vi "Post action control.vi"(1 "Action":u16(ring)=4 items=["Clear DAQ Tasks", "Check Temperature", "Check Field Value", "Wait", "Do Nothing"], 2 "Scan Parameters":T1={"DAQ Channel"=1, "Label"="\nappliedVsg=", "Scaled low"=-0.1, "Scaled high"=0.1, "Start"=-0.32, "End"=0.42, "Step"=0.002, "Scale?"=FALSE} {"Step" format="%#_6p"; "End" format="%#_6p"; "Start" format="%#_6p"; "Scaled high" format="%#_6p"; "Scaled low" format="%#_6p"}, 3 "Index":dbl=370.0) -> (0 "Out":u16(ring)=4 items=["Clear DAQ Tasks", "Check Temperature", "Check Field Value", "Do Nothing"])   [LabVIEW 2013]
uses:
  <userlib>/LevyLab/PPMS_VIs/Lockin-4461_MultiChannel - IV 3.0 globals.vi
panel:
  in  "target temperature":dbl=0.07
  in  "milliseconds to wait":u32=5000
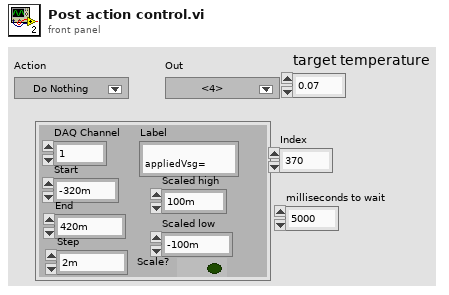
[diagram p1: front panel]
types:
  T1 = cluster{"DAQ Channel":i32, "Label":string, "Scaled low":dbl, "Scaled high":dbl, "Start":dbl, "End":dbl, "Step":dbl, "Scale?":bool}
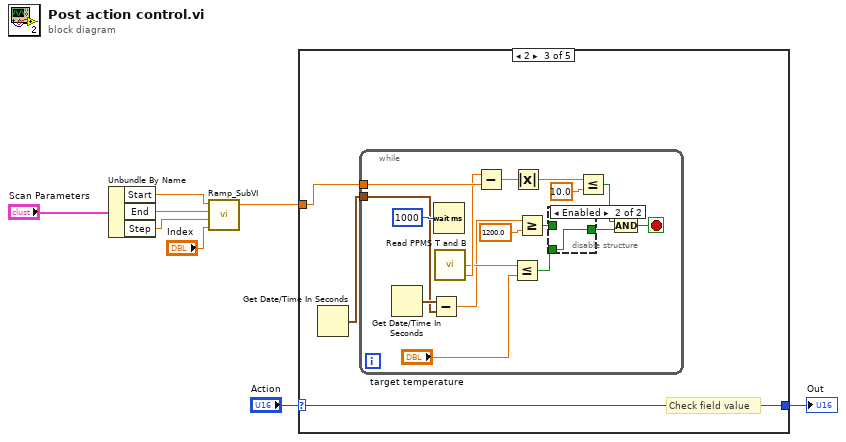
[diagram p0: block diagram]
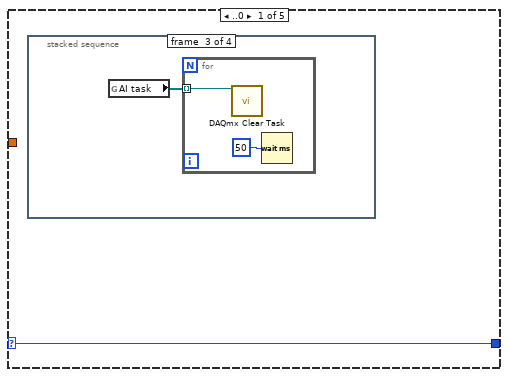
[diagram p2: hidden frame]
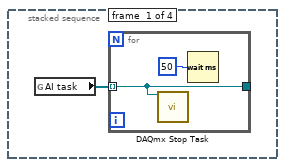
[diagram p3: hidden frame]
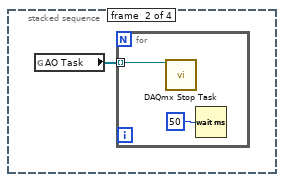
[diagram p4: hidden frame]
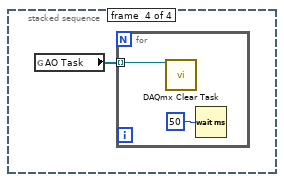
[diagram p5: hidden frame]
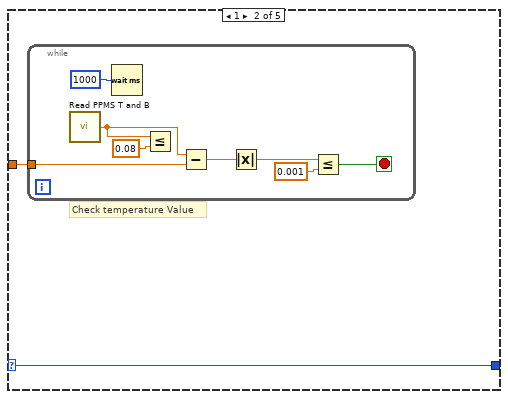
[diagram p6: hidden frame]
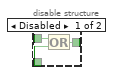
[diagram p7: hidden frame]
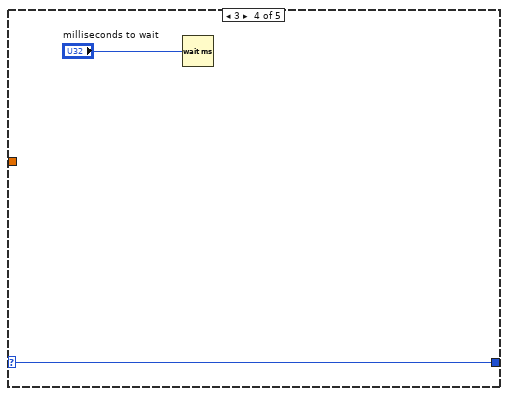
[diagram p8: hidden frame]
diagram:
  n1 = Unbundle By Name("Scan Parameters") -> ("Start"=w5:dbl, "End"=w4:dbl, "Step"=w3:dbl)
  n2 = call <userlib>:"Ramp_SubVI.vi"("index"="Index", "step"=w3, "end"=w4, "start"=w5) -> ("Numeric"=w7:dbl)  [unwired: 1 in, 1 out]
  n3 = case shown="2" "Action" {
    tunnel: w7 -> [_ w23 w34 _ _]
    selector: "Action" -> [w9 w22 w33 w57 w58]
    tunnel: [w9 w22 w33 w57 w58] -> w1
    frame ..0 {
      n4 = stacked-sequence {
        frame #0 {
          n5 = global read "Lockin-4461_MultiChannel - IV 3.0 globals.vi" "AI task"() -> (w10:refnum<k21>[])
          n6 = for {
            tunnel: w10 -> [w11] mode=indexing
            tunnel: [w11] -> _
            n7 = call <vilib>:"DAQmx Stop Task.vi"("task/channels in"=w11) -> ()  [unwired: 13 in, 2 out]
            n8 = Wait (ms)(milliseconds to wait=u32 50) -> ()  [unwired: 1 out]
          }
        }
        frame #1 {
          n9 = global read "Lockin-4461_MultiChannel - IV 3.0 globals.vi" "AO Task"() -> (w13:refnum<k21>[])
          n10 = for {
            tunnel: w13 -> [w15] mode=indexing
            n11 = call <vilib>:"DAQmx Stop Task.vi"("task/channels in"=w15) -> ()  [unwired: 13 in, 2 out]
            n12 = Wait (ms)(milliseconds to wait=u32 50) -> ()  [unwired: 1 out]
          }
        }
        frame #2 {
          n13 = global read "Lockin-4461_MultiChannel - IV 3.0 globals.vi" "AI task"() -> (w16:refnum<k21>[])
          n14 = for {
            tunnel: w16 -> [w18] mode=indexing
            n15 = call <vilib>:"DAQmx Clear Task.vi"("task in"=w18) -> ()  [unwired: 14 in, 1 out]
            n16 = Wait (ms)(milliseconds to wait=u32 50) -> ()  [unwired: 1 out]
          }
        }
        frame #3 {
          n17 = global read "Lockin-4461_MultiChannel - IV 3.0 globals.vi" "AO Task"() -> (w19:refnum<k21>[])
          n18 = for {
            tunnel: w19 -> [w21] mode=indexing
            n19 = call <vilib>:"DAQmx Clear Task.vi"("task in"=w21) -> ()  [unwired: 14 in, 1 out]
            n20 = Wait (ms)(milliseconds to wait=u32 50) -> ()  [unwired: 1 out]
          }
        }
      }
    }
    frame 1 {
      # "Check temperature Value"
      n21 = while {
        tunnel: w23 -> [w27]
        stop <- w24 stop-if-true
        n22 = call "Read PPMS T and B.vi"() -> ("Temperature"=w26:dbl)  [unwired: 3 in, 2 out]
        n23 = Wait (ms)(milliseconds to wait=u32 1000) -> ()  [unwired: 1 out]
        n24 = Less Or Equal?(x=w26, y=0.08) -> ()  [unwired: 1 out]
        n25 = Subtract(x=w26, y=w27) -> (x-y=w31:dbl)
        n26 = Absolute Value(x=w31) -> (abs(x)=w30:dbl)
        n27 = Less Or Equal?(x=w30, y=0.001) -> (x <= y?=w24:bool)
      }
    }
    frame 2 {
      # "Check field value"
      n28 = Get Date/Time In Seconds() -> (seconds since 1Jan1904=w32:timestamp)
      n29 = while {
        tunnel: w34 -> [w51]
        tunnel: w32 -> [w40]
        stop <- w42 stop-if-true
        n30 = Get Date/Time In Seconds() -> (seconds since 1Jan1904=w41:timestamp)
        n31 = Subtract(x=w41, y=w40) -> (x-y=w39:dbl)
        n32 = Wait (ms)(milliseconds to wait=u32 1000) -> ()  [unwired: 1 out]
        n33 = call "Read PPMS T and B.vi"() -> ("Field"=w46:dbl, "Temperature"=w44:dbl)  [unwired: 3 in, 1 out]
        n34 = Subtract(x=w46, y=w51) -> (x-y=w50:dbl)
        n35 = Less Or Equal?(x=w44, y="target temperature") -> (x <= y?=w37:bool)
        n36 = Absolute Value(x=w50) -> (abs(x)=w49:dbl)
        n37 = Greater Or Equal?(x=w39, y=1200.0) -> (x >= y?=w36:bool)
        n38 = disable-structure shown="Enabled" {
          disable-tunnel: w37 -> [w54 w55]
          disable-tunnel: w36 -> [w53 _]
          disable-tunnel: [w52 w55] -> w35
          frame Disabled {
            n39 = Or(x=w53, y=w54) -> (x .or. y?=w52:bool)
          }
          frame Enabled {
          }
        }
        n40 = Less Or Equal?(x=w49, y=10.0) -> (x <= y?=w43:bool)
        n41 = And(x=w43, y=w35) -> (x .and. y?=w42:bool)
      }
    }
    frame 3 {
      n42 = Wait (ms)(milliseconds to wait="milliseconds to wait") -> ()  [unwired: 1 out]
    }
    frame 4.. {
      # "Do nothing"
    }
  }
  "Out" <- w1
